vi "Mind Read.vi"() -> ()   [LabVIEW 2014]
uses:
  <vilib>/Utility/error.llb/DialogType.ctl
  <vilib>/NI/LabVIEW - NeuroSky Driver/NeuroSky Driver/ThinkGear Read/ThinkGear MultiSample Read Raw.vi
  <vilib>/NI/LabVIEW - NeuroSky Driver/NeuroSky Driver.lvlib
panel:
  in  "Stop Button":bool
  out "1":bool
  out "2":bool
  out "3":bool
  out "4":bool
  out "5":bool
  out "Raw EEG Signal":sgl[](graph)
  # "Monitor panels"
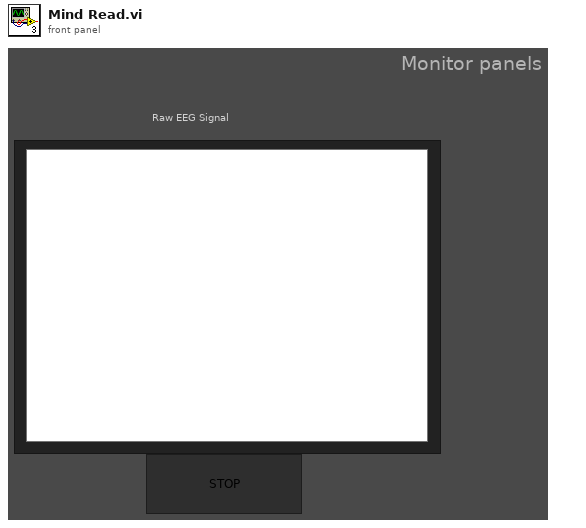
[diagram p1: front panel]
types:
  T1 = typedef "DialogType.ctl" = u16
  T2 = cluster{"connectionId":i32, "serialPortName":string, "serialBaudrate":i32, "serialDataFormat":i32}
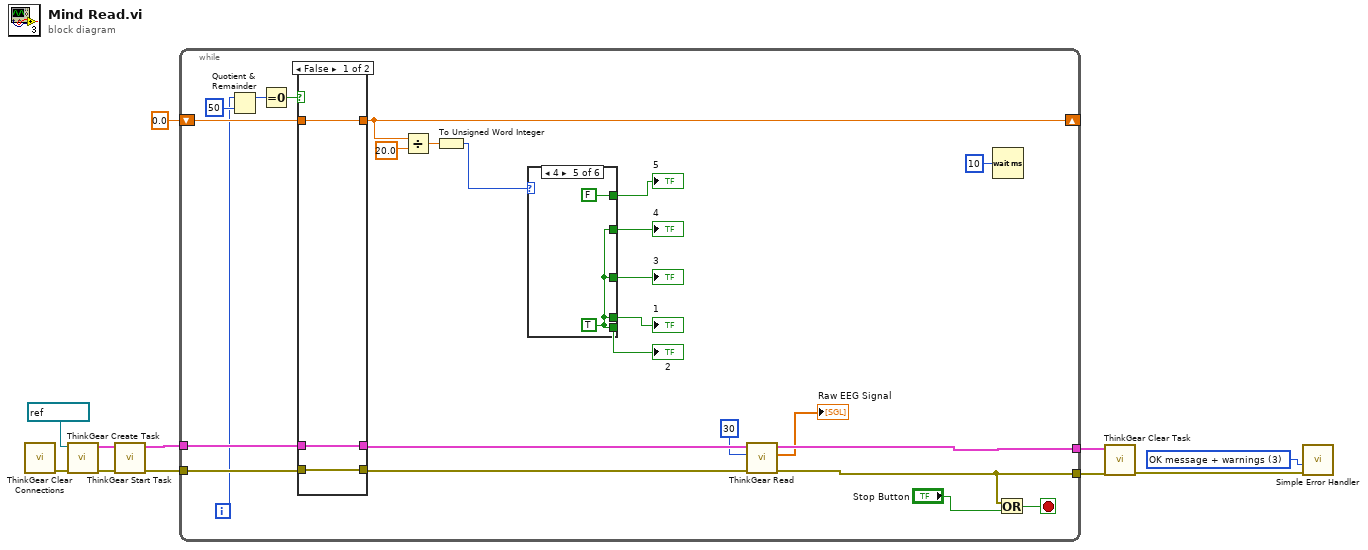
[diagram p0: block diagram]
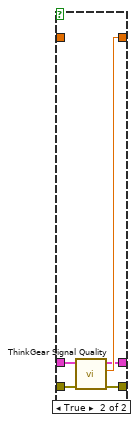
[diagram p2: hidden frame]
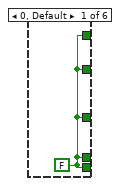
[diagram p3: hidden frame]
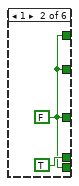
[diagram p4: hidden frame]
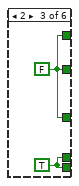
[diagram p5: hidden frame]
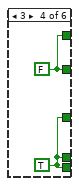
[diagram p6: hidden frame]
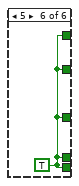
[diagram p7: hidden frame]
diagram:
  w11 = T1 3 items=["no dialog", "OK message", "continue or stop message", "OK message + warnings", "continue/stop + warnings"] ("type of dialog (OK msg:1)")
  n1 = call <vilib>:"ThinkGear Clear Connections.vi"() -> ("error out"=w9:errorcluster)  [unwired: 11 in]
  n2 = call <vilib>:"ThinkGear Create Task.vi"("error in"=w9, "serialPortName"=refnum<visa-resource-name> "COM6") -> ("error out"=w2:errorcluster, "NeuroSky Task Out"=w1:T2)  [unwired: 8 in]
  n3 = call <vilib>:"ThinkGear Start Task.vi"("error in (no error)"=w2, "NeuroSky Task In"=w1) -> ("error out"=w7:errorcluster, "NeuroSky Task Out"=w8:T2)  [unwired: 8 in]
  n4 = while {
    tunnel: w8 -> [w34]
    tunnel: w7 -> [w35]
    shift-right: [w24] -> _
    shift-left: sgl 0.0 ("y") -> [w25]
    tunnel: [w17] -> w4
    tunnel: [w16] -> w3
    i -> [w15]
    stop <- w36 stop-if-true
    n5 = Quotient & Remainder(x=w15, y=50) -> (x-y*floor(x/y)=w22:i32)  [unwired: 1 out]
    n6 = Equal To 0?(x=w22) -> (x = 0?=w21:bool)
    n7 = case shown="False" w21 {
      tunnel: w35 -> [w38 w44]
      tunnel: w34 -> [w39 w40]
      tunnel: [w37 w43] -> w24
      tunnel: [w38 w42] -> w20
      tunnel: [w39 w41] -> w19
      tunnel: w25 -> [w37 _]
      frame False {
      }
      frame True {
        n8 = call <vilib>:"ThinkGear Signal Quality.vi"("error in (no error)"=w44, "NeuroSky Task In"=w40) -> ("error out"=w42:errorcluster, "Signal Quality"=w43:sgl, "NeuroSky Task Out"=w41:T2)  [unwired: 7 in]
      }
    }
    n9 = Divide(x=w24, y=sgl 20.0) -> (x/y=w31:sgl)
    n10 = To Unsigned Word Integer(number=w31) -> (unsigned 16bit integer=w32:u16)
    n11 = case shown="4" w32 {
      tunnel: [w45 TRUE w48 w50 w52 w54] -> w30
      tunnel: [w45 w46 w48 w50 w52 w54] -> w29
      tunnel: [w45 w46 w49 w50 w52 w54] -> w28
      tunnel: [w45 w46 w49 w51 w52 w54] -> w27
      tunnel: [w45 w46 w49 w51 FALSE w54] -> w26
      frame 0, Default {
        w45 = FALSE
      }
      frame 1 {
        w46 = FALSE
      }
      frame 2 {
        w49 = FALSE
        w48 = TRUE
      }
      frame 3 {
        w51 = FALSE
        w50 = TRUE
      }
      frame 4 {
        w52 = TRUE
      }
      frame 5 {
        w54 = TRUE
      }
    }
    "1" <- w30
    "2" <- w29
    "3" <- w28
    "4" <- w27
    "5" <- w26
    n12 = call-poly <vilib>:"ThinkGear Read.vi"("error in (no error)"=w20, "Samples to Read"=30, "NeuroSky Task In"=w19) -> ("error out"=w16:errorcluster, "Data Out"=→"Raw EEG Signal":sgl[], "NeuroSky Task Out"=w17:T2)  [unwired: 6 in]
    n13 = Wait (ms)(milliseconds to wait=u32 10) -> ()  [unwired: 1 out]
    n14 = Or(x=w16, y="Stop Button") -> (x .or. y?=w36:bool)
  }
  n15 = call <vilib>:"ThinkGear Clear Task.VI"("error in"=w3, "NeuroSky Task In"=w4) -> ("error out"=w10:errorcluster)  [unwired: 9 in]
  n16 = call <vilib>:"Simple Error Handler.vi"("type of dialog (OK msg:1)"=w11, "error in (no error)"=w10) -> ()  [unwired: 3 in, 5 out]
